vi "StartUp Sequence Open Loop Rev 1.6.vi"() -> ()   [LabVIEW 2017]
uses:
  <vilib>/addons/control/pid/pid.llb/PID (DBL).vi
  <vilib>/addons/control/pid/NI_PID_pid.lvlib
panel:
  out "Process variable and Setpoint":cluster{i32, "Requested RPM:":dbl}(graph)
  in  "PID gains":T1={"proportional gain (Kc)"=1.0, "integral time (Ti, min)"=0.0, "derivative time (Td, min)"=0.0} {"derivative time (Td, min)" format="%.3f"; "integral time (Ti, min)" format="%.3f"; "proportional gain (Kc)" format="%.3f"}
  out "Measured RPM (thousands):":dbl(slide)=60.754431603254424 scale=44.0..130.0
  in  "Requested RPM (thousands):":dbl(slide)=45.0 min=0.0 max=0.0 scale=44.0..130.0
  out "MV:":dbl(slide)=18.78965245852964 scale=80.0..150.0
  out "Manipulated variable":dbl(graph)
  out "Waveform Chart":cluster{i32, "Requested RPM (thousands):":dbl}(graph)
  out "Pump Value 2":string
  in  "Soft Shut Off":bool
  out "Pump Value 1":string
  in  "Send Command":bool
  in  "Custom Command":string
  out "Startup Success":bool
  in  "Output File":path
  in  "Shut Off":bool
  out "ECU COM Port Out":refnum<visa-resource-name>
  out "Throttle Position":string
  out "Turbine RPM":string
  out "Turbine Temp":string
  out "Error Out":errorcluster
  in  "Error In":errorcluster
  in  "ECU COM Port":refnum<visa-resource-name>
  out "Turbine State":string
  in  "Strt Sqnc":bool
  # "Note: save to a .csv file"
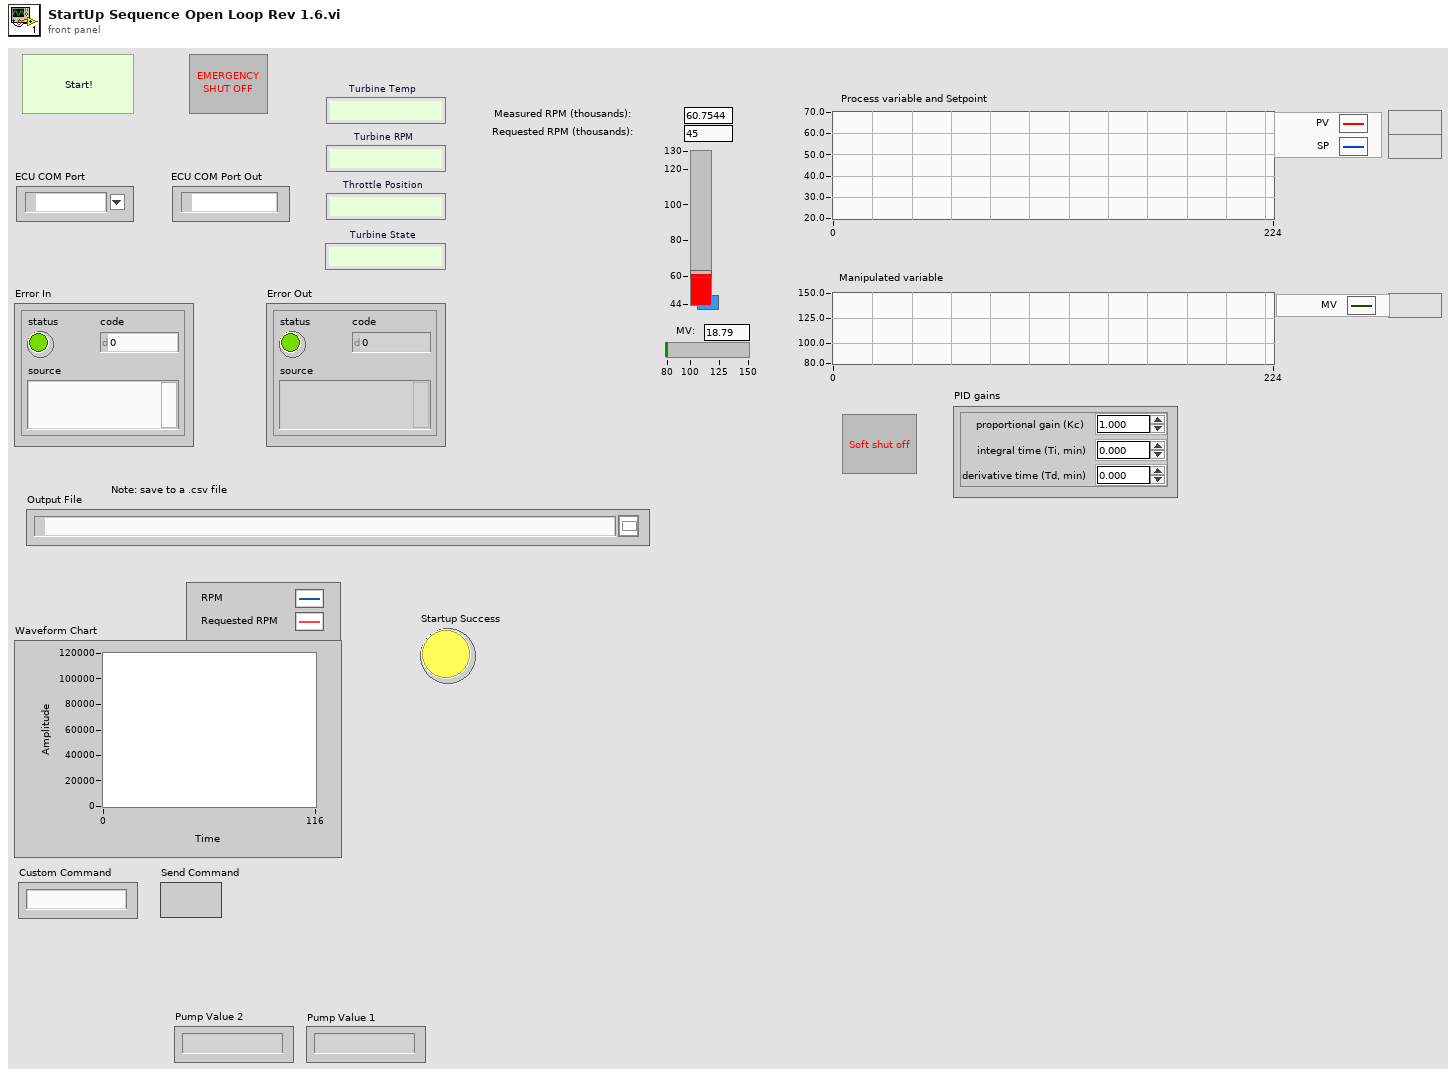
[diagram p1: front panel]
types:
  T1 = cluster{"proportional gain (Kc)":dbl, "integral time (Ti, min)":dbl, "derivative time (Td, min)":dbl}
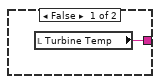
[diagram p3: hidden frame]
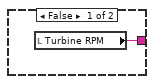
[diagram p4: hidden frame]
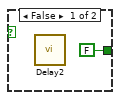
[diagram p7: hidden frame]
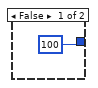
[diagram p8: hidden frame]
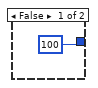
[diagram p9: hidden frame]
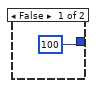
[diagram p10: hidden frame]
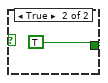
[diagram p11: hidden frame]
diagram:
  w18 = 21 ("Pulse Width")
  w19 = 160 ("Voltage")
  w24 = 16 ("Pulse Width")
  w25 = 160 ("Voltage")
  w15 = 255 ("y")
  w16 = 80 ("y")
  # "Disengage Starter Motor"
  # "Starter Motor 55%"
  # "Start button is inside a while loop that doesn't progess until True"
  # "Fuel Pump Mode 2"
  # "GlowPlugOff"
  # "Start Up\nFuelPumpMode 1"
  # "BurnerValveIgnitionPercent"
  # "If False, each Case structure is set\nto an arbitrary Delay time of 0.2 s"
  # "Each Stage is inside a while loop so that \nthe sequence doesn't progress until True"
  n1 = call "Initialize Com Port.vi"("Error In"="Error In", "ECU COM Port"="ECU COM Port") -> ("Error Out"=w35:errorcluster, "ECU COM Port Out"=w34:refnum<visa-resource-name>)  [unwired: 8 in]
  n2 = while {
    tunnel: w35 -> [w97]
    tunnel: [w97] -> w33
    stop <- "Strt Sqnc" stop-if-true
  }
  n3 = call "Initialize Output File.vi"("error in (no error)"=w33, "File Path Control"="Output File") -> ("error out"=w14:errorcluster)  [unwired: 9 in]
  n4 = flat-sequence {
    tunnel: w14 -> [w99]
    tunnel: [w99] -> w29
    frame #0 {
      n5 = local write "Strt Sqnc"(FALSE ("Strt Sqnc")) -> ()
    }
  }
  n6 = flat-sequence {
    tunnel: [w102] -> w13
    tunnel: w14 -> [w102]
    frame #0 {
      w101 = "0" ("Pump Value 1")
      n7 = local write "Pump Value 2"(w101) -> ()
      n8 = local write "Pump Value 1"(w101) -> ()
    }
  }
  n9 = while {
    tunnel: w13 -> [w125]
    tunnel: w34 -> [w124]
    tunnel: "Output File" -> [w121]
    stop <- w120 continue-if-true
    n10 = call "Get Engine Update.vi"("Error In"=w125, "ECU COM Port"=w124) -> ("Error Out"=w122:errorcluster, "Temperature"=w113:string, "RPMs"=w117:string, "ECU COM Port Out"=w119:refnum<visa-resource-name>)  [unwired: 6 in]
    n11 = call "Time Delay4"() -> ()  [unwired: 11 in, 1 out]
    n12 = call "Safety Check.vi"("Temperature"=w113, "RPMs"=w117) -> ("Safe?"=w120:bool)  [unwired: 9 in]
    n13 = Not Equal?(x=w117, y="") -> (x != y?=w115:bool)
    n14 = Not Equal?(x=w113, y="") -> (x != y?=w112:bool)
    n15 = case shown="False" w120 {
      selector: w120 -> [w130 w132]
      tunnel: w119 -> [w131 _]
      tunnel: [w130 w132] -> w118
      frame False {
        n16 = call "Emergency Shutoff.vi"("ECU COM Port"=w131) -> ()  [unwired: 9 in, 2 out]
      }
      frame True {
      }
    }
    n17 = case shown="True" w115 {
      tunnel: w117 -> [_ w129]
      tunnel: [w128 w129] -> w109
      frame False {
        n18 = local read "Turbine RPM"() -> (w128:string)
      }
      frame True {
        "Turbine RPM" <- w129
      }
    }
    n19 = case shown="True" w112 {
      tunnel: w113 -> [_ w127]
      tunnel: [w126 w127] -> w108
      frame False {
        n20 = local read "Turbine Temp"() -> (w126:string)
      }
      frame True {
        "Turbine Temp" <- w127
      }
    }
    n21 = Not(x=w118) -> (.not. x?=w123:bool)
    n22 = Stop(stop? (T)=w123) -> ()
    n23 = local read "Requested RPM (thousands):"() -> (w104:dbl)
    n24 = local read "Pump Value 2"() -> (w110:string)
    n25 = local read "Pump Value 1"() -> (w111:string)
    n26 = Decimal String To Number(string=w109) -> (number=w107:i32)  [unwired: 2 in, 1 out]
    n27 = Multiply(x=w104, y=1000.0) -> (x*y=w105:dbl)
    n28 = Bundle(w107, w105) -> (→"Waveform Chart":cluster{i32, dbl})  [unwired: 1 in]
    n29 = call "Write Data to Output File.vi"("Pump Value 2"=w110, "Pump Value 1"=w111, "Error In"=w122, "Temperature"=w108, "RPM"=w109, "File Path Control"=w121) -> ()  [unwired: 5 in, 1 out]
  }
  n30 = while {
    tunnel: w34 -> [w134]
    tunnel: w35 -> [_]
    stop <- FALSE stop-if-true
    n31 = case shown="True" "Send Command" {
      tunnel: "Custom Command" -> [_ w138]
      tunnel: w134 -> [_ w137]
      frame False {
      }
      frame True {
        n32 = call "Time Delay3"() -> ()  [unwired: 11 in, 1 out]
        n33 = VISA Write(VISA resource name=w137, write buffer=w138) -> ()  [unwired: 1 in, 3 out]
      }
    }
  }
  n34 = flat-sequence {
    tunnel: w29 -> [_]
    frame #0 {
      n35 = local write "Turbine State"("Initializing Motor") -> ()
    }
  }
  n36 = while {
    tunnel: ["Shut Off"] -> w94
    tunnel: "ECU COM Port" -> [w140]
    stop <- "Shut Off" stop-if-true
    # "Turns off each individual component"
    n37 = case shown="True" "Shut Off" {
      tunnel: w140 -> [_ w144]
      frame False {
      }
      frame True {
        n38 = call "Emergency Shutoff.vi"("ECU COM Port"=w144) -> ("Error Out"=w143:errorcluster)  [unwired: 9 in, 1 out]
        n39 = local write "Output File"(path "" ("Output File")) -> ()
        n40 = flat-sequence {
          tunnel: w143 -> [w145]
          tunnel: [w145] -> _
          frame #0 {
            n41 = local write "Strt Sqnc"(FALSE ("Strt Sqnc")) -> ()
          }
        }
      }
    }
  }
  n42 = call "Set Glow Plug Duty Cycle.vi"("Error In"=w29, "Duty Cycle"=6, "ECU COM Port"=w34) -> ("Error Out"=w86:errorcluster, "ECU COM Port Out"=w83:refnum<visa-resource-name>)  [unwired: 7 in]
  n43 = call "Delay"("error in (no error)"=w86) -> ("error out"=w85:errorcluster)  [unwired: 10 in]
  n44 = call "Set Glow Plug Duty Cycle.vi"("Error In"=w85, "Duty Cycle"=19, "ECU COM Port"=w83) -> ("Error Out"=w84:errorcluster, "ECU COM Port Out"=w79:refnum<visa-resource-name>)  [unwired: 7 in]
  n45 = call "Delay"("error in (no error)"=w84) -> ("error out"=w80:errorcluster)  [unwired: 10 in]
  n46 = call "Set Starter Motor Duty Cycle.vi"("Error In"=w80, "Duty Cycle"=6, "ECU COM Port"=w79) -> ("Error Out"=w78:errorcluster, "ECU COM Port Out"=w76:refnum<visa-resource-name>)  [unwired: 7 in]
  n47 = call "Set Glow Plug Duty Cycle.vi"("Error In"=w78, "Duty Cycle"=15, "ECU COM Port"=w76) -> ("Error Out"=w77:errorcluster, "ECU COM Port Out"=w72:refnum<visa-resource-name>)  [unwired: 7 in]
  n48 = call "Delay"("error in (no error)"=w77) -> ("error out"=w74:errorcluster)  [unwired: 10 in]
  n49 = call "Set Starter Motor Duty Cycle.vi"("Error In"=w74, "Duty Cycle"=4, "ECU COM Port"=w72) -> ("Error Out"=w73:errorcluster, "ECU COM Port Out"=w71:refnum<visa-resource-name>)  [unwired: 7 in]
  n50 = call "Delay"("error in (no error)"=w73) -> ("error out"=w95:errorcluster)  [unwired: 10 in]
  n51 = Stop(stop? (T)=w94) -> ()
  n52 = while {
    tunnel: w95 -> [w149]
    tunnel: w71 -> [w148]
    tunnel: [w148] -> w27
    tunnel: [w149] -> w96
    stop <- w152 stop-if-true
    n53 = local read "Turbine RPM"() -> (w147:string)
    n54 = Decimal String To Number(string=w147) -> (number=w151:i32)  [unwired: 2 in, 1 out]
    n55 = Greater Or Equal?(x=w151, y=3300) -> (x >= y?=w153:bool)
    n56 = case shown="True" w153 {
      tunnel: [FALSE TRUE] -> w152
      frame False {
        n57 = call "Delay2"() -> ()  [unwired: 11 in, 1 out]
      }
      frame True {
      }
    }
  }
  n58 = flat-sequence {
    tunnel: w95 -> [_]
    frame #0 {
      n59 = local write "Turbine State"("Stage1 Check RPM") -> ()
    }
  }
  n60 = call "CmdSeparator7"("error in (no error)"=w96) -> ("error out"=w23:errorcluster)  [unwired: 10 in]
  n61 = call "Set Pump Fow Rate.vi"("Error In"=w23, "Pulse Width"=w24, "Voltage"=w25, "ECU COM Port"=w27) -> ("Error Out"=w28:errorcluster, "ECU COM Port Out"=w26:refnum<visa-resource-name>)  [unwired: 6 in]
  n62 = flat-sequence {
    tunnel: w25 -> [w158]
    tunnel: w24 -> [w157]
    tunnel: w23 -> [_]
    frame #0 {
      n63 = Number To Decimal String(number=w157) -> (decimal integer string=w159:string)  [unwired: 1 in]
      n64 = Number To Decimal String(number=w158) -> (decimal integer string=w160:string)  [unwired: 1 in]
      n65 = local write "Pump Value 2"(w159) -> ()
      n66 = local write "Pump Value 1"(w160) -> ()
    }
  }
  n67 = call "CmdSeparator2"("error in (no error)"=w28) -> ("error out"=w70:errorcluster)  [unwired: 10 in]
  n68 = call "Set Burner Valve Percent.vi"("Error In"=w70, "Percent"=10, "ECU COM Port"=w26) -> ("Error Out"=w2:errorcluster, "ECU COM Port Out"=w5:refnum<visa-resource-name>)  [unwired: 7 in]
  n69 = call "CmdSeparator4"("error in (no error)"=w2) -> ("error out"=w1:errorcluster)  [unwired: 10 in]
  n70 = for {
    N: 8 -> [_]
    shift-right: [w166] -> _
    shift-left: 27 ("Percent") -> [w168]
    tunnel: w5 -> [w165]
    tunnel: w1 -> [w164]
    tunnel: [w162] -> w3
    tunnel: [w161] -> w4
    n71 = Add(x=w168, y=4 ("Percent")) -> (x+y=w166:i32)
    n72 = call "Set Burner Valve Percent.vi"("Error In"=w164, "Percent"=w166, "ECU COM Port"=w165) -> ("Error Out"=w163:errorcluster, "ECU COM Port Out"=w161:refnum<visa-resource-name>)  [unwired: 7 in]
    n73 = call "CmdSeparator"("error in (no error)"=w163) -> ("error out"=w162:errorcluster)  [unwired: 10 in]
  }
  n74 = flat-sequence {
    tunnel: w3 -> [_]
    frame #0 {
      n75 = local write "Turbine State"("Stage2 Check Temp.") -> ()
    }
  }
  n76 = while {
    tunnel: w4 -> [w171]
    tunnel: w3 -> [w172]
    tunnel: [w171] -> w64
    tunnel: [w172] -> w65
    stop <- w175 stop-if-true
    # "Stage2Temp(C)"
    n77 = local read "Turbine Temp"() -> (w170:string)
    n78 = Decimal String To Number(string=w170) -> (number=w173:i32)  [unwired: 2 in, 1 out]
    n79 = Greater Or Equal?(x=w173, y=90) -> (x >= y?=w176:bool)
    n80 = case shown="False" w176 {
      tunnel: [FALSE TRUE] -> w175
      frame False {
        n81 = call "Delay3"() -> ()  [unwired: 11 in, 1 out]
      }
      frame True {
      }
    }
  }
  n82 = call "Set Glow Plug Duty Cycle.vi"("Error In"=w65, "Duty Cycle"=0, "ECU COM Port"=w64) -> ("Error Out"=w63:errorcluster, "ECU COM Port Out"=w20:refnum<visa-resource-name>)  [unwired: 7 in]
  n83 = call "CmdSeparator3"("error in (no error)"=w63) -> ("error out"=w17:errorcluster)  [unwired: 10 in]
  n84 = call "Set Pump Fow Rate.vi"("Error In"=w17, "Pulse Width"=w18, "Voltage"=w19, "ECU COM Port"=w20) -> ("Error Out"=w22:errorcluster, "ECU COM Port Out"=w21:refnum<visa-resource-name>)  [unwired: 6 in]
  n85 = call "Set Burner Valve Percent.vi"("Error In"=w22, "Percent"=80, "ECU COM Port"=w21) -> ("Error Out"=w60:errorcluster, "ECU COM Port Out"=w61:refnum<visa-resource-name>)  [unwired: 7 in]
  n86 = flat-sequence {
    tunnel: w19 -> [w180]
    tunnel: w18 -> [w179]
    tunnel: w17 -> [_]
    frame #0 {
      n87 = Number To Decimal String(number=w179) -> (decimal integer string=w181:string)  [unwired: 1 in]
      n88 = Number To Decimal String(number=w180) -> (decimal integer string=w182:string)  [unwired: 1 in]
      n89 = local write "Pump Value 2"(w181) -> ()
      n90 = local write "Pump Value 1"(w182) -> ()
    }
  }
  n91 = call "CmdSeparator18"("error in (no error)"=w60) -> ("error out"=w59:errorcluster)  [unwired: 10 in]
  n92 = call "Set Fuel Valve Percent.vi"("Error In"=w59, "Percent"=12, "ECU COM Port"=w61) -> ("Error Out"=w58:errorcluster, "ECU COM Port Out"=w62:refnum<visa-resource-name>)  [unwired: 7 in]
  n93 = call "CmdSeparator16"("error in (no error)"=w58) -> ("error out"=w92:errorcluster)  [unwired: 10 in]
  n94 = for {
    N: 4 -> [_]
    tunnel: [w183] -> _
    tunnel: [w197] -> _
    tunnel: w62 -> [w189]
    tunnel: w92 -> [w190]
    shift-right: [w188] -> w54
    shift-left: 12 -> [w194]
    shift-right: [w185] -> _
    shift-left: 80 -> [w191]
    tunnel: [w197] -> w49 mode=indexing
    tunnel: [w183] -> w55 mode=indexing
    n95 = Less?(x=w194, y=100) -> (x < y?=w195:bool)
    n96 = Less?(x=w191, y=100) -> (x < y?=w192:bool)
    n97 = case shown="True" w192 {
      tunnel: w191 -> [_ w201]
      tunnel: [100 w199] -> w185
      frame False {
      }
      frame True {
        n98 = Add(x=w201, y=5) -> (x+y=w199:i32)
      }
    }
    n99 = case shown="True" w195 {
      tunnel: w194 -> [_ w205]
      tunnel: [100 w203] -> w188
      frame False {
      }
      frame True {
        n100 = Add(x=w205, y=6) -> (x+y=w203:i32)
      }
    }
    n101 = call "Set Fuel Valve Percent.vi"("Error In"=w190, "Percent"=w188, "ECU COM Port"=w189) -> ("Error Out"=w187:errorcluster, "ECU COM Port Out"=w184:refnum<visa-resource-name>)  [unwired: 7 in]
    n102 = call "Set Burner Valve Percent.vi"("Error In"=w187, "Percent"=w185, "ECU COM Port"=w184) -> ("Error Out"=w186:errorcluster, "ECU COM Port Out"=w183:refnum<visa-resource-name>)  [unwired: 7 in]
    n103 = call "CmdSeparator17"("error in (no error)"=w186) -> ("error out"=w197:errorcluster)  [unwired: 10 in]
  }
  n104 = flat-sequence {
    tunnel: w49 -> [_]
    frame #0 {
      n105 = local write "Turbine State"("Pump Ramp Up") -> ()
    }
  }
  n106 = for {
    N: 10 -> [_]
    tunnel: [w213] -> w37
    tunnel: [w224] -> w40
    shift-right: [w220] -> _
    shift-left: w54 -> [w221]
    tunnel: w49 -> [w217] mode=indexing
    tunnel: w55 -> [w216] mode=indexing
    shift-right: [w209] -> w51
    shift-left: 21 -> [w210]
    w208 = 160 ("y")
    n107 = Less?(x=w221, y=100) -> (x < y?=w222:bool)
    n108 = Add(x=w210, y=1) -> (x+y=w209:i32)
    n109 = case shown="True" w222 {
      tunnel: w221 -> [_ w232]
      tunnel: [100 w230] -> w220
      frame False {
      }
      frame True {
        n110 = Add(x=w232, y=5) -> (x+y=w230:i32)
      }
    }
    n111 = call "Set Fuel Valve Percent.vi"("Error In"=w217, "Percent"=w220, "ECU COM Port"=w216) -> ("Error Out"=w219:errorcluster, "ECU COM Port Out"=w218:refnum<visa-resource-name>)  [unwired: 7 in]
    n112 = call "Set Burner Valve Percent.vi"("Error In"=w219, "Percent"=100 ("y"), "ECU COM Port"=w218) -> ("Error Out"=w207:errorcluster, "ECU COM Port Out"=w214:refnum<visa-resource-name>)  [unwired: 7 in]
    n113 = call "Set Pump Fow Rate.vi"("Error In"=w207, "Pulse Width"=w209, "Voltage"=w208, "ECU COM Port"=w214) -> ("Error Out"=w212:errorcluster, "ECU COM Port Out"=w213:refnum<visa-resource-name>)  [unwired: 6 in]
    n114 = flat-sequence {
      tunnel: w208 -> [w226]
      tunnel: w209 -> [w225]
      tunnel: w207 -> [_]
      frame #0 {
        n115 = Number To Decimal String(number=w225) -> (decimal integer string=w227:string)  [unwired: 1 in]
        n116 = Number To Decimal String(number=w226) -> (decimal integer string=w228:string)  [unwired: 1 in]
        n117 = local write "Pump Value 2"(w227) -> ()
        n118 = local write "Pump Value 1"(w228) -> ()
      }
    }
    n119 = call "CmdSeparator20"("error in (no error)"=w212) -> ("error out"=w224:errorcluster)  [unwired: 10 in]
  }
  n120 = call "Set Starter Motor Duty Cycle.vi"("Error In"=w40, "Duty Cycle"=11, "ECU COM Port"=w37) -> ("Error Out"=w39:errorcluster, "ECU COM Port Out"=w38:refnum<visa-resource-name>)  [unwired: 7 in]
  n121 = flat-sequence {
    tunnel: w39 -> [_]
    frame #0 {
      n122 = local write "Turbine State"("Secondary Pump Ramp Up") -> ()
    }
  }
  n123 = for {
    N: 3 -> [_]
    tunnel: [w241] -> w50
    tunnel: [w248] -> w48
    tunnel: w39 -> [w245]
    tunnel: w38 -> [w244]
    shift-right: [w235] -> _
    shift-left: w51 -> [w238]
    w236 = 160 ("y")
    n124 = Add(x=w238, y=10) -> (x+y=w235:i32)
    n125 = call "Set Fuel Valve Percent.vi"("Error In"=w245, "Percent"=100 ("y"), "ECU COM Port"=w244) -> ("Error Out"=w247:errorcluster, "ECU COM Port Out"=w246:refnum<visa-resource-name>)  [unwired: 7 in]
    n126 = call "Set Burner Valve Percent.vi"("Error In"=w247, "Percent"=0 ("y"), "ECU COM Port"=w246) -> ("Error Out"=w234:errorcluster, "ECU COM Port Out"=w242:refnum<visa-resource-name>)  [unwired: 7 in]
    n127 = call "Set Pump Fow Rate.vi"("Error In"=w234, "Pulse Width"=w235, "Voltage"=w236, "ECU COM Port"=w242) -> ("Error Out"=w240:errorcluster, "ECU COM Port Out"=w241:refnum<visa-resource-name>)  [unwired: 6 in]
    n128 = flat-sequence {
      tunnel: w236 -> [w250]
      tunnel: w235 -> [w249]
      tunnel: w234 -> [_]
      frame #0 {
        n129 = Number To Decimal String(number=w249) -> (decimal integer string=w251:string)  [unwired: 1 in]
        n130 = Number To Decimal String(number=w250) -> (decimal integer string=w252:string)  [unwired: 1 in]
        n131 = local write "Pump Value 2"(w251) -> ()
        n132 = local write "Pump Value 1"(w252) -> ()
      }
    }
    n133 = call "CmdSeparator15"("error in (no error)"=w240) -> ("error out"=w248:errorcluster)  [unwired: 10 in]
  }
  n134 = flat-sequence {
    tunnel: w48 -> [_]
    frame #0 {
      n135 = local write "Turbine State"("Hold on to your butts!") -> ()
    }
  }
  n136 = while {
    tunnel: w48 -> [w255]
    tunnel: w50 -> [w254]
    tunnel: [w255] -> w12
    tunnel: [w254] -> w47
    stop <- w256 stop-if-true
    n137 = local read "Turbine RPM"() -> (w259:string)
    n138 = Decimal String To Number(string=w259) -> (number=w258:i32)  [unwired: 2 in, 1 out]
    n139 = Greater?(x=w258, y=30000) -> (0:w256:bool)
  }
  n140 = call "Set Pump Fow Rate.vi"("Error In"=w12, "Pulse Width"=w15, "Voltage"=w16, "ECU COM Port"=w47) -> ("Error Out"=w46:errorcluster, "ECU COM Port Out"=w45:refnum<visa-resource-name>)  [unwired: 6 in]
  n141 = flat-sequence {
    tunnel: w16 -> [w262]
    tunnel: w15 -> [w261]
    tunnel: [w260] -> _
    tunnel: w12 -> [w260]
    frame #0 {
      n142 = Number To Decimal String(number=w261) -> (decimal integer string=w263:string)  [unwired: 1 in]
      n143 = Number To Decimal String(number=w262) -> (decimal integer string=w264:string)  [unwired: 1 in]
      n144 = local write "Pump Value 2"(w263) -> ()
      n145 = local write "Pump Value 1"(w264) -> ()
    }
  }
  n146 = while {
    tunnel: w46 -> [w266]
    tunnel: w45 -> [w265]
    tunnel: [w266] -> w42
    tunnel: [w265] -> w44
    stop <- w267 stop-if-true
    n147 = local read "Turbine RPM"() -> (w270:string)
    n148 = Decimal String To Number(string=w270) -> (number=w269:i32)  [unwired: 2 in, 1 out]
    n149 = Greater?(x=w269, y=44000) -> (0:w267:bool)
  }
  n150 = flat-sequence {
    tunnel: w42 -> [_]
    frame #0 {
      n151 = local write "Turbine State"("Acheived Idle RPM!") -> ()
    }
  }
  n152 = call "Set Starter Motor Duty Cycle.vi"("Error In"=w42, "Duty Cycle"=0, "ECU COM Port"=w44) -> ("Error Out"=w10:errorcluster, "ECU COM Port Out"=w11:refnum<visa-resource-name>)  [unwired: 7 in]
  n153 = flat-sequence {
    tunnel: w10 -> [_]
    frame #0 {
      "Startup Success" <- TRUE
    }
  }
  n154 = while {
    tunnel: [w284] -> w9
    tunnel: [w283] -> w8
    tunnel: w11 -> [w281]
    tunnel: w10 -> [w282]
    stop <- "Soft Shut Off" stop-if-true
    # "Control loop using PID"
    n155 = local read "Turbine RPM"() -> (w280:string)
    n156 = Decimal String To Number(string=w280) -> (number=w276:i32)  [unwired: 2 in, 1 out]
    n157 = Divide(x=w276, y=1000) -> (x/y=w273:dbl)
    "Measured RPM (thousands):" <- w273
    n158 = Wait Until Next ms Multiple(millisecond multiple=u32 500 ("unsigned 32bit integer")) -> ()  [unwired: 1 out]
    n159 = call-poly <vilib>:"PID.vi"("output range"=cluster{"output high":dbl, "output low":dbl} {"output high"=100.0, "output low"=80.0}, "PID gains"="PID gains", "process variable"=w273, "setpoint"="Requested RPM (thousands):") -> ("output"=w278:dbl)  [unwired: 6 in, 1 out]
    "MV:" <- w278
    "Manipulated variable" <- w278
    n160 = Bundle(w276, "Requested RPM (thousands):"="Requested RPM (thousands):") -> (→"Process variable and Setpoint":cluster{i32, "Requested RPM (thousands):":dbl})  [unwired: 1 in]
    n161 = Number To Decimal String(number=w278) -> (decimal integer string=→"Pump Value 1":string)  [unwired: 1 in]
    n162 = call "Set Pump Fow Rate.vi"("Error In"=w282, "Pulse Width"=255, "Voltage"=w278, "ECU COM Port"=w281) -> ("Error Out"=w283:errorcluster, "ECU COM Port Out"=w284:refnum<visa-resource-name>)  [unwired: 6 in]
    n163 = local write "Pump Value 2"("255" ("Pump Value 2")) -> ()
  }
  n164 = call "Emergency Shutoff.vi"("Error In"=w8, "ECU COM Port"=w9) -> ("Error Out"=w31:errorcluster, "ECU COM Port Out"=→"ECU COM Port Out":refnum<visa-resource-name>)  [unwired: 8 in]
  n165 = flat-sequence {
    tunnel: w31 -> [w292]
    tunnel: [w292] -> w93
    frame #0 {
      w291 = "0"
      n166 = local write "Pump Value 1"(w291) -> ()
      n167 = local write "Pump Value 2"(w291) -> ()
    }
  }
  "Error Out" <- w93
